vi "Trajectory_Sample.vi"(9 "Time":dbl, 11 "InputTRAJECTORY":T5 {"TotalTImeSecs" format="%20.3f"}) -> (3 "OutputTRAJ_STATE":T1={"TimeSeconds"=0.0, "Velocity"=0.0, "Acceleration"=0.0, "POSE"={"TRANSLATION"={"X"=0.0, "Y"=0.0}, "ROTATION"={"VALUE"=0.0, "COS"=1.0, "SIN"=0.0}}, "Curvature"=0.0})   [LabVIEW 2019, in "Trajectory_Library.lvlib"]
doc: "Sample the trajectory at a point in time.\n \nParameters:\n - InputTrajectory - The Trajectory data structure\n - time - The point in time since the beginning of the trajectory to sample. (seconds)\n\nReturns:\n - OutputTrajState - The state at that point in time."
uses:
  TRAJECTORY.ctl
  TRAJ_STATE.ctl
  POSE2D.ctl
  TRANSLATION2D.ctl
  ROTATION2D.ctl
  Trajectory_Library.lvlib
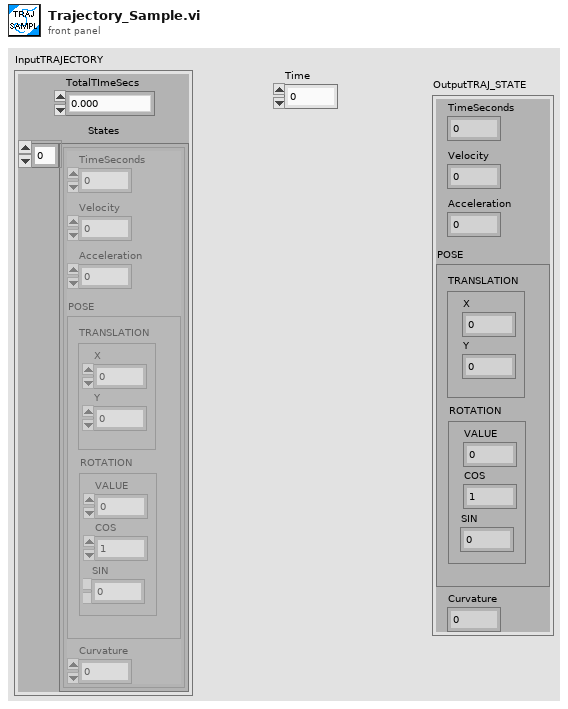
[diagram p1: front panel]
types:
  T1 = typedef "Trajectory_Library.lvlib/TRAJ_STATE.ctl" = cluster{"TimeSeconds":dbl, "Velocity":dbl, "Acceleration":dbl, "POSE":T2, "Curvature":dbl}
  T2 = typedef "Trajectory_Library.lvlib/POSE2D.ctl" = cluster{"TRANSLATION":T3, "ROTATION":T4}
  T3 = typedef "Trajectory_Library.lvlib/TRANSLATION2D.ctl" = cluster{"X":dbl, "Y":dbl}
  T4 = typedef "Trajectory_Library.lvlib/ROTATION2D.ctl" = cluster{"VALUE":dbl, "COS":dbl, "SIN":dbl}
  T5 = typedef "Trajectory_Library.lvlib/TRAJECTORY.ctl" = cluster{"TotalTImeSecs":dbl, "States":T1[]}
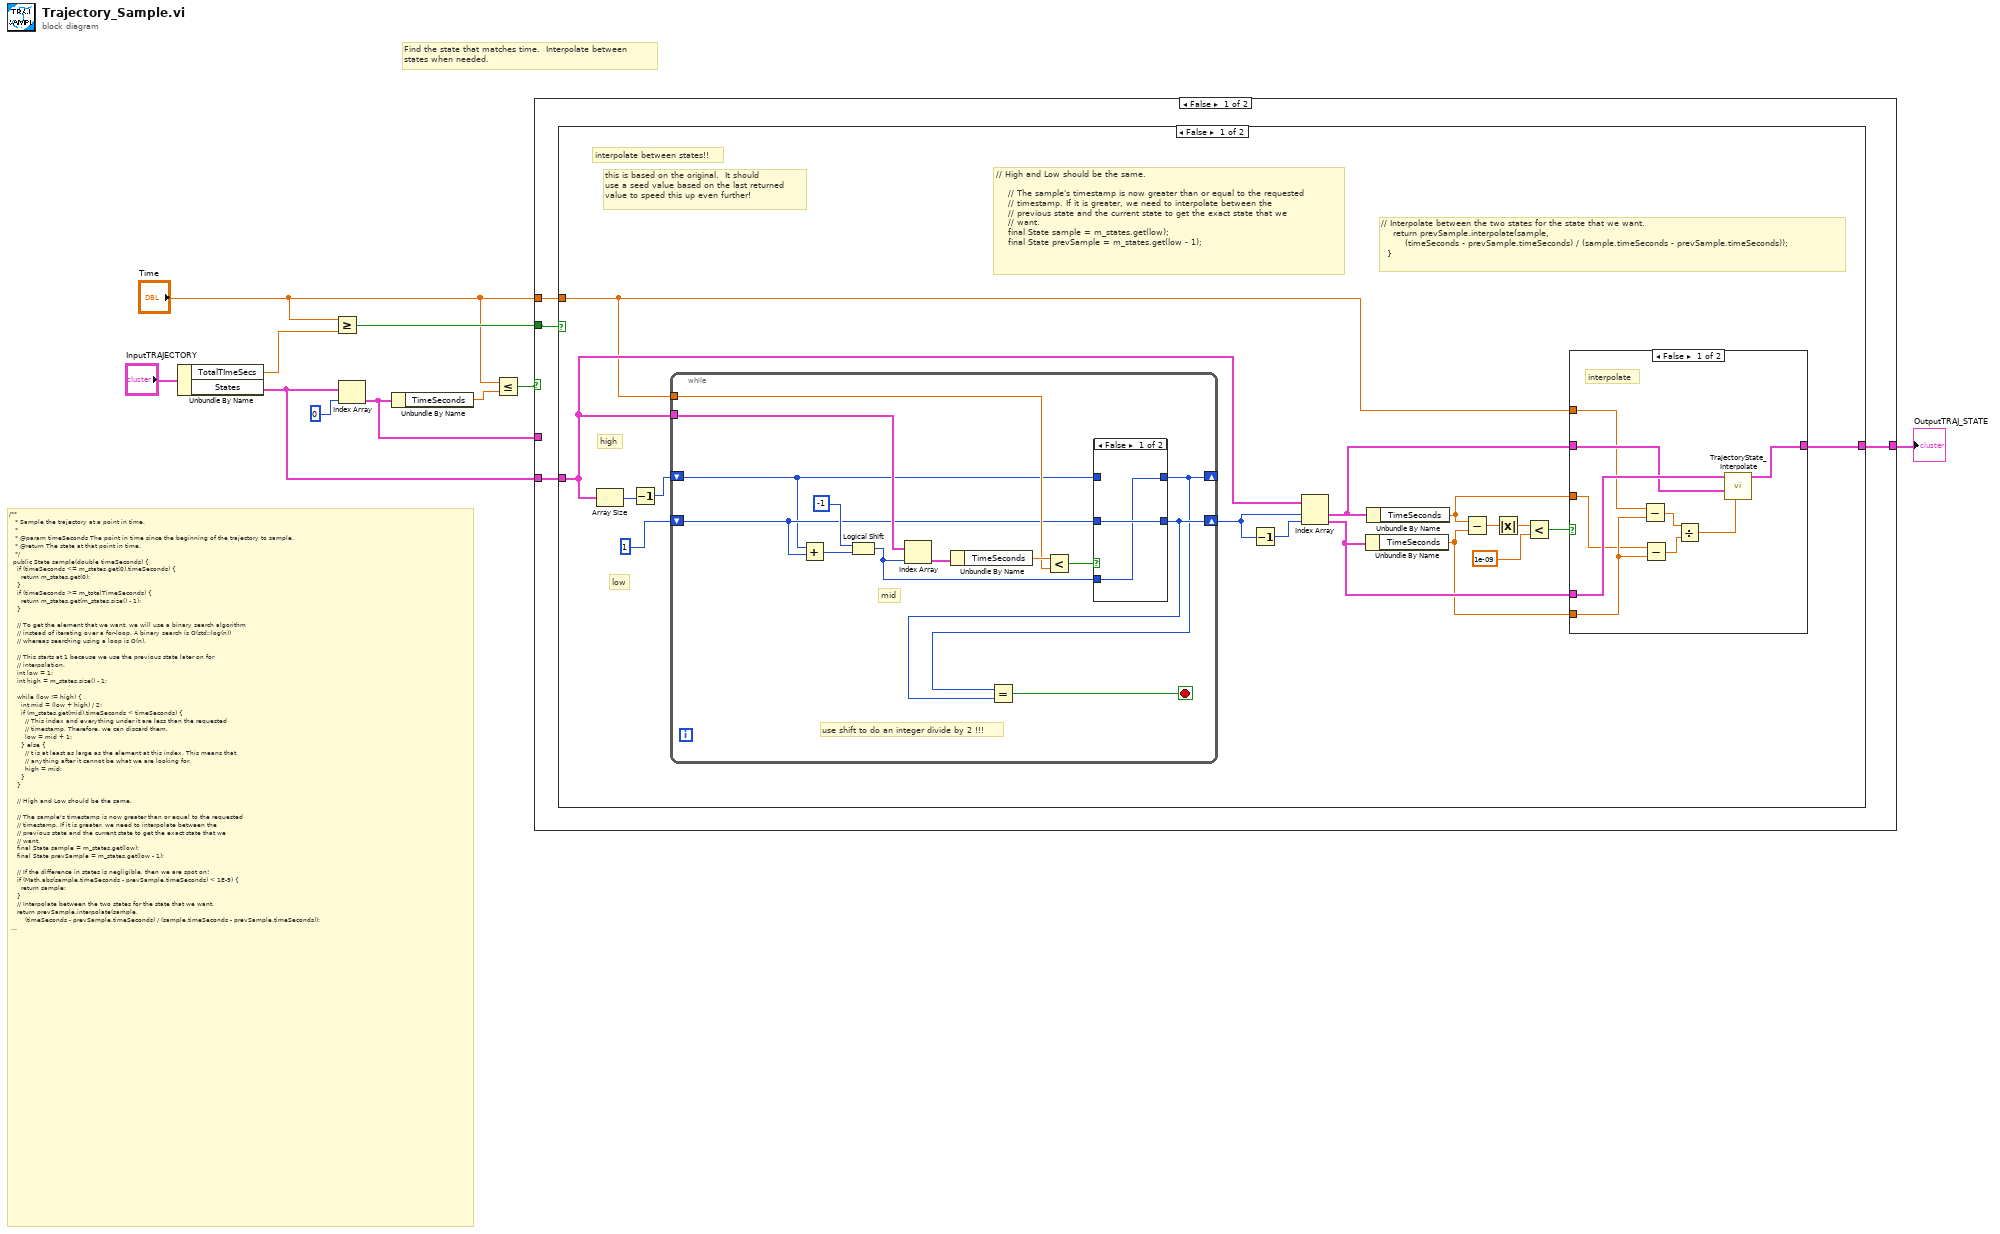
[diagram p0: block diagram]
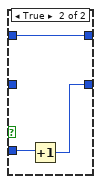
[diagram p3: hidden frame]
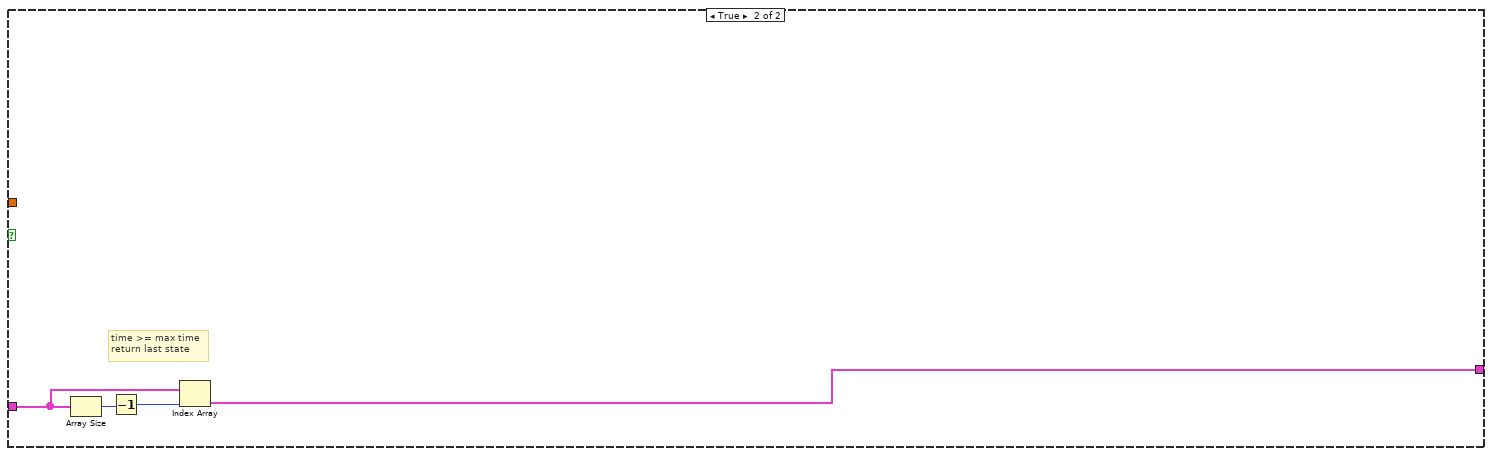
[diagram p4: hidden frame]
diagram:
  # "/**\n   * Sample the trajectory at a point in time.\n   *\n   * @param timeSeconds The point in time since the beginning of the trajectory to sample.\n   * @return The state at that point in time.\n   */\n  public State sample(double timeSeconds) {\n    if (timeSeconds <= m_states.get(0).timeSeconds) {\n      return m_states.get(0);\n    }\n    if (timeSeconds >= m_totalTimeSeconds) {\n      return m_states.get(m_states.size() - 1);\n    }\n\n    // To get the element that we want, we will use a binary search algorithm\n    // instead of iterating over a for-loop. A binary search is O(std::log(n))\n    // whereas searching using a loop is O(n).\n\n    // This starts at 1 because we use the previous state later on for\n    // interpolation.\n    int low = 1;\n    int high = m_states.size() - 1;\n\n    while (low != high) {\n      int mid = (low + high) / 2;\n      if (m_states.get(mid).timeSeconds < timeSeconds) {\n        // This index and everything under it are less than the requested\n        // timestamp. Therefore, we can discard them.\n        low = mid + 1;\n      } else {\n        // t is at least as large as the element at this index. This means that\n        // anything after it cannot be what we are looking for.\n        high = mid;\n      }\n    }\n\n    // High and Low should be the same.\n\n    // The sample's timestamp is now greater than or equal to the requested\n    // timestamp. If it is greater, we need to interpolate between the\n    // previous state and the current state to get the exact state that we\n    // want.\n    final State sample = m_states.get(low);\n    final State prevSample = m_states.get(low - 1);\n\n    // If the difference in states is negligible, then we are spot on!\n    if (Math.abs(sample.timeSeconds - prevSample.timeSeconds) < 1E-9) {\n      return sample;\n    }\n    // Interpolate between the two states for the state that we want.\n    return prevSample.interpolate(sample,\n        (timeSeconds - prevSample.timeSeconds) / (sample.timeSeconds - prevSample.timeSeconds));\n  }"
  # "Find the state that matches time.  Interpolate between\nstates when needed."
  n1 = Unbundle By Name("InputTRAJECTORY") -> ("TotalTImeSecs"=w8:dbl, "States"=w2:T1[])
  n2 = Greater Or Equal?(x="Time", y=w8) -> (x >= y?=w3:bool)
  n3 = Index Array(array=w2, index=0) -> (element=w5:T1)
  n4 = Unbundle By Name(w5) -> ("TimeSeconds"=w7:dbl)
  n5 = Less Or Equal?(x="Time", y=w7) -> (x <= y?=w6:bool)
  n6 = case shown="False" w6 {
    tunnel: w5 -> [_ w63]
    tunnel: [w12 w63] -> w4
    tunnel: w3 -> [w14 _]
    tunnel: w2 -> [w13 _]
    tunnel: "Time" -> [w11 _]
    frame False {
      n7 = case shown="False" w14 {
        tunnel: w13 -> [w29 w60]
        tunnel: [w21 w59] -> w12
        tunnel: w11 -> [w19 _]
        frame False {
          # "// Interpolate between the two states for the state that we want.\n    return prevSample.interpolate(sample,\n        (timeSeconds - prevSample.timeSeconds) / (sample.timeSeconds - prevSample.timeSeconds));\n  }"
          # "// High and Low should be the same.\n\n    // The sample's timestamp is now greater than or equal to the requested\n    // timestamp. If it is greater, we need to interpolate between the\n    // previous state and the current state to get the exact state that we\n    // want.\n    final State sample = m_states.get(low);\n    final State prevSample = m_states.get(low - 1);"
          # "this is based on the original.  It should\nuse a seed value based on the last returned\nvalue to speed this up even further!"
          # "low"
          # "high"
          # "interpolate between states!!"
          n8 = Array Size(array=w29) -> (size(s)=w30:i32)
          n9 = Decrement(x=w30) -> (x-1=w16:i32)
          n10 = while {
            shift-right: [w45] -> _
            shift-left: w16 -> [w41]
            shift-right: [w46] -> w28
            shift-left: 1 -> [w42]
            tunnel: w29 -> [w52]
            tunnel: w19 -> [w48]
            stop <- w53 stop-if-true
            # "use shift to do an integer divide by 2 !!!"
            # "mid"
            n11 = Add(x=w41, y=w42) -> (x+y=w44:i32)
            n12 = Logical Shift(y=-1, x=w44) -> (x << y=w47:i32)
            n13 = Index Array(array=w52, index=w47) -> (element=w51:T1)
            n14 = Unbundle By Name(w51) -> ("TimeSeconds"=w50:dbl)
            n15 = Less?(x=w50, y=w48) -> (x < y?=w49:bool)
            n16 = case shown="False" w49 {
              tunnel: w41 -> [_ w58]
              tunnel: [w54 w58] -> w45
              tunnel: w42 -> [w55 _]
              tunnel: w47 -> [w54 w57]
              tunnel: [w55 w56] -> w46
              frame False {
              }
              frame True {
                n17 = Increment(x=w57) -> (x+1=w56:i32)
              }
            }
            n18 = Equal?(x=w45, y=w46) -> (x = y?=w53:bool)
          }
          n19 = Decrement(x=w28) -> (x-1=w27:i32)
          n20 = Index Array(array=w29, index #1=w28, index #2=w27) -> (element #1=w22:T1, element #2=w20:T1)
          n21 = Unbundle By Name(w20) -> ("TimeSeconds"=w18:dbl)
          n22 = Unbundle By Name(w22) -> ("TimeSeconds"=w17:dbl)
          n23 = Subtract(x=w17, y=w18) -> (x-y=w26:dbl)
          n24 = Absolute Value(x=w26) -> (abs(x)=w25:dbl)
          n25 = Less?(x=w25, y=1e-09) -> (x < y?=w23:bool)
          n26 = case shown="False" w23 {
            tunnel: w22 -> [w38 w40]
            tunnel: [w31 w40] -> w21
            tunnel: w20 -> [w39 _]
            tunnel: w19 -> [w37 _]
            tunnel: w18 -> [w36 _]
            tunnel: w17 -> [w35 _]
            frame False {
              # "interpolate"
              n27 = Subtract(x=w37, y=w36) -> (x-y=w33:dbl)
              n28 = Subtract(x=w35, y=w36) -> (x-y=w34:dbl)
              n29 = Divide(x=w33, y=w34) -> (x/y=w32:dbl)
              n30 = call "TrajectoryState_Interpolate.vi"("interpolantFraction"=w32, "endValueTRAJ_STATE"=w38, "inputTRAJ_STATE"=w39) -> ("OutputTRAJ_STATE"=w31:T1)  [unwired: 8 in]
            }
            frame True {
              # "both the same"
            }
          }
        }
        frame True {
          # "time >= max time\nreturn last state"
          n31 = Array Size(array=w60) -> (size(s)=w62:i32)
          n32 = Decrement(x=w62) -> (x-1=w61:i32)
          n33 = Index Array(array=w60, index=w61) -> (element=w59:T1)
        }
      }
    }
    frame True {
      # "time <= first time\nreturn first state"
    }
  }
  "OutputTRAJ_STATE" <- w4
